vi "Draw.vi"(11 "Yeld":dbl) -> (3 "2D Picture":picture)   [LabVIEW 2019, in "TestBench.lvlib" / "TestBench.lvclass"]
uses:
  TestBench.lvclass
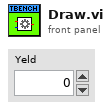
[diagram p1: front panel]
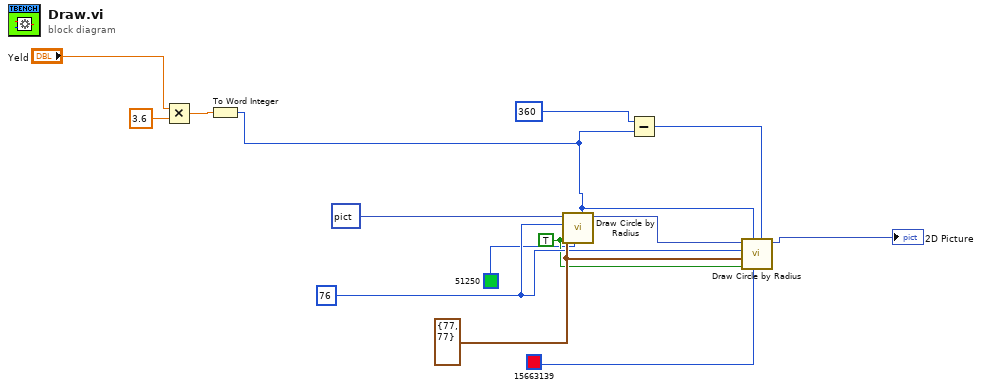
[diagram p0: block diagram]
diagram:
  w13 = cluster{"horizontal":i16, "vertical":i16} {"horizontal"=77, "vertical"=77} ("pixel center")
  w8 = TRUE ("fill?(F)")
  w12 = i16 76 ("radius")
  n1 = Multiply(x="Yeld", y=3.6) -> (x*y=w2:dbl)
  n2 = To Word Integer(number=w2) -> (16bit integer=w1:i16)
  n3 = call <vilib>:"Draw Circle by Radius.vi"("arc size(360)"=w1, "color(black)"=u32 51250, "fill?(F)"=w8, "pixel center"=w13, "radius"=w12, "picture"=picture data[5B]) -> ("new picture"=w14:picture)  [unwired: 5 in]
  n4 = Subtract(x=i16 360 ("arc size(360)"), y=w1) -> (x-y=w9:i16)
  n5 = call <vilib>:"Draw Circle by Radius.vi"("arc size(360)"=w9, "color(black)"=u32 15663139 ("color(black) 2"), "start angle(0)"=w1, "fill?(F)"=w8, "pixel center"=w13, "radius"=w12, "picture"=w14) -> ("new picture"=→"2D Picture":picture)  [unwired: 4 in]
